vi "MasaDelSol.vi"() -> ()   [LabVIEW 2018]
panel:
  out "Masa del Sol":dbl
  in  "Distancia Tierra al Sol":dbl=149600000000.0
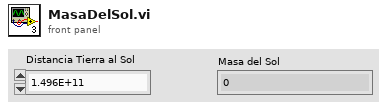
[diagram p1: front panel]
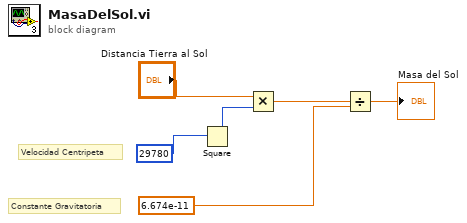
[diagram p0: block diagram]
diagram:
  # "Constante Gravitatoria"
  # "Velocidad Centripeta"
  n1 = Square(x=29780) -> (x^2=w4:i32)
  n2 = Multiply(x="Distancia Tierra al Sol", y=w4) -> (x*y=w5:dbl)
  n3 = Divide(x=w5, y=6.674e-11) -> (x/y=→"Masa del Sol":dbl)
